vi "setupDevPopulateTree.vi"(8 "error in (no error)":errorcluster, 9 "Elternobjekt-Tag":string, 10 "TreeControl in":refnum<vi>, 11 "used devices":refnum<class "Device.lvclass">[](array[class])) -> (0 "error out":errorcluster, 2 "#dev":i32)   [LabVIEW 2013, in "DataCreation.lvlib"]
uses:
  DataCreation.lvlib
  classes/Datastructure/Device/Device.lvclass
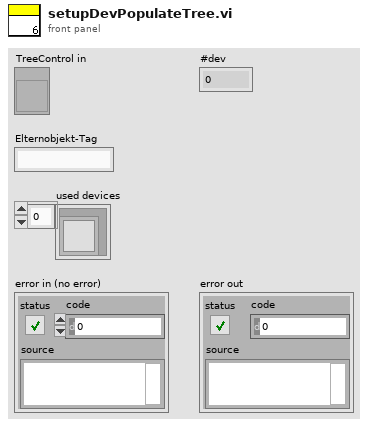
[diagram p1: front panel]
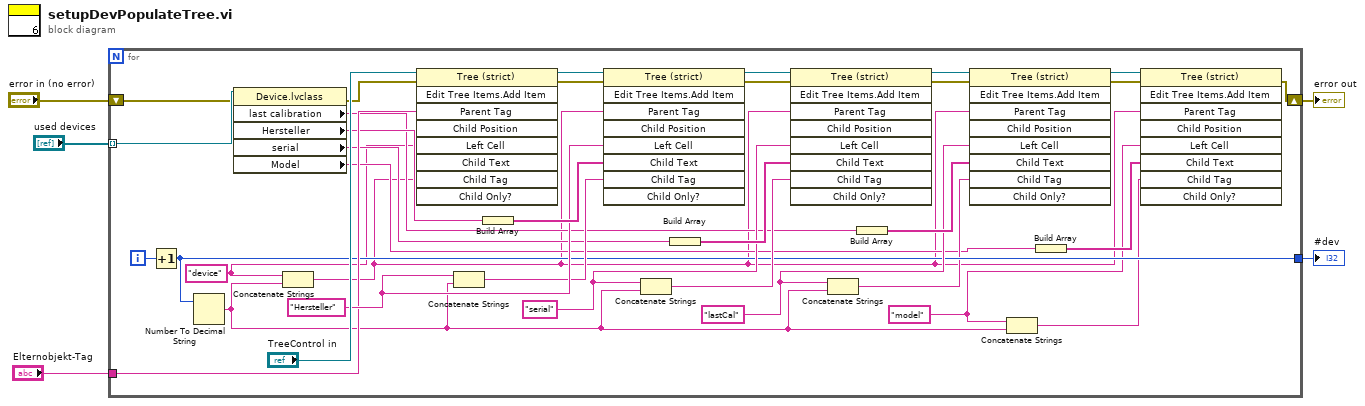
[diagram p0: block diagram]
diagram:
  n1 = for {
    tunnel: "used devices" -> [w24] mode=indexing
    tunnel: "Elternobjekt-Tag" -> [w25]
    shift-right: [w10] -> w3
    shift-left: "error in (no error)" -> [w23]
    tunnel: [w17] -> w5
    i -> [w18]
    w9 = "model" ("Linker Zellen-String")
    w26 = "lastCal" ("Linker Zellen-String")
    w28 = "serial" ("Linker Zellen-String")
    w30 = "Hersteller" ("Linker Zellen-String")
    w7 = "device" ("Left Cell String")
    n2 = Increment(x=w18) -> (x+1=w17:i32)
    n3 = Number To Decimal String(number=w17) -> (decimal integer string=w6:string)  [unwired: 1 in]
    n4 = property class="Device.lvclass"(reference=w24, error in=w23) -> (error out=w22:errorcluster, "last calibration"=w19:string, "Hersteller"=w21:string, "serial"=w20:string, "Model"=w12:string)  [unwired: 1 out]
    n5 = Concatenate Strings(w7, w6) -> (w8:string)
    n6 = invoke class="Tree (strict)" method="Edit Tree Items.Add Item"(reference="TreeControl in", error in=w22, "Parent Tag"=w25, "Left Cell"=w7, "Child Tag"=w8) -> (reference out=w38:refnum<vi>, error out=w39:errorcluster)  [unwired: 4 in, 7 out]
    n7 = Concatenate Strings(w30, w6) -> (w29:string)
    n8 = Build Array(w21) -> (w33:string[])
    n9 = invoke class="Tree (strict)" method="Edit Tree Items.Add Item"(reference=w38, error in=w39, "Parent Tag"=w8, "Left Cell"=w30, "Child Text"=w33, "Child Tag"=w29) -> (reference out=w37:refnum<vi>, error out=w36:errorcluster)  [unwired: 3 in, 7 out]
    n10 = Concatenate Strings(w28, w6) -> (w27:string)
    n11 = Build Array(w20) -> (w32:string[])
    n12 = invoke class="Tree (strict)" method="Edit Tree Items.Add Item"(reference=w37, error in=w36, "Parent Tag"=w8, "Left Cell"=w28, "Child Text"=w32, "Child Tag"=w27) -> (reference out=w34:refnum<vi>, error out=w35:errorcluster)  [unwired: 3 in, 7 out]
    n13 = Concatenate Strings(w26, w6) -> (w14:string)
    n14 = Build Array(w19) -> (w31:string[])
    n15 = invoke class="Tree (strict)" method="Edit Tree Items.Add Item"(reference=w34, error in=w35, "Parent Tag"=w8, "Left Cell"=w26, "Child Text"=w31, "Child Tag"=w14) -> (reference out=w16:refnum<vi>, error out=w15:errorcluster)  [unwired: 3 in, 7 out]
    n16 = Concatenate Strings(w9, w6) -> (w13:string)
    n17 = Build Array(w12) -> (w11:string[])
    n18 = invoke class="Tree (strict)" method="Edit Tree Items.Add Item"(reference=w16, error in=w15, "Parent Tag"=w8, "Left Cell"=w9, "Child Text"=w11, "Child Tag"=w13) -> (error out=w10:errorcluster)  [unwired: 3 in, 8 out]
  }
  "#dev" <- w5
  "error out" <- w3
